vi "XW_Type_1b_correction.vi"(1 "variable n":bool, 2 "wire diameter (mu.m)":dbl, 3 "calib consts. t2":dbl[](array[numeric]), 4 "calib consts. t1":dbl[](array[numeric])) -> (0 "Corrected calib consts. t2":dbl[](array[numeric]))   [LabVIEW 2011]
panel:
  # "Type 1b: Correct calibration constants at t2 to conditions at t1"
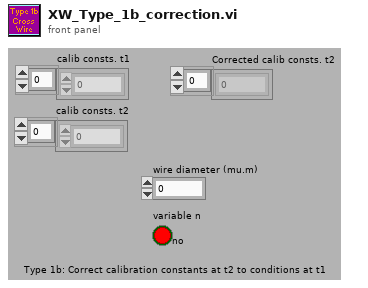
[diagram p1: front panel]
types:
  T1 = cluster{"calib consts. t1[0]":dbl, "calib consts. t1[1]":dbl, "calib consts. t1[2]":dbl, "calib consts. t1[3]":dbl, "calib consts. t1[4]":dbl, "calib consts. t1[5]":dbl, "calib consts. t1[6]":dbl, "calib consts. t1[7]":dbl, "calib consts. t1[8]":dbl, "calib consts. t1[9]":dbl, "calib consts. t1[10]":dbl, "calib consts. t1[11]":dbl, "calib consts. t1[12]":dbl, "calib consts. t1[13]":dbl, "calib consts. t1[14]":dbl, "calib consts. t1[15]":dbl, "calib consts. t1[16]":dbl, "calib consts. t1[17]":dbl}
  T2 = cluster{"calib consts. t2[0]":dbl, "calib consts. t2[1]":dbl, "calib consts. t2[2]":dbl, "calib consts. t2[3]":dbl, "calib consts. t2[4]":dbl, "calib consts. t2[5]":dbl, "calib consts. t2[6]":dbl, "calib consts. t2[7]":dbl, "calib consts. t2[8]":dbl, "calib consts. t2[9]":dbl, "calib consts. t2[10]":dbl, "calib consts. t2[11]":dbl, "calib consts. t2[12]":dbl, "calib consts. t2[13]":dbl, "calib consts. t2[14]":dbl, "calib consts. t2[15]":dbl, "calib consts. t2[16]":dbl, "calib consts. t2[17]":dbl}
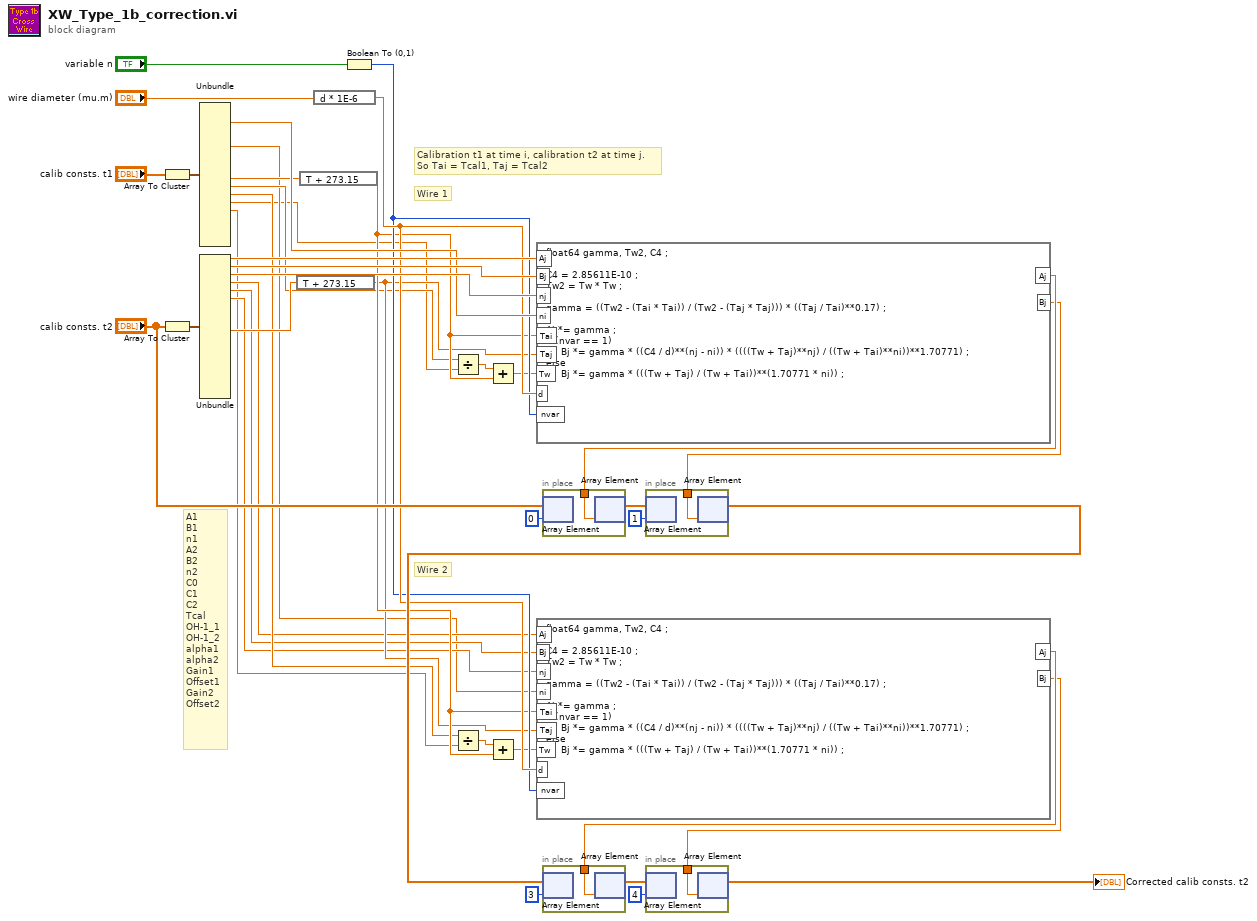
[diagram p0: block diagram]
diagram:
  # "Wire 2"
  # "Wire 1"
  # "A1\nB1\nn1\nA2\nB2\nn2\nC0\nC1\nC2\nTcal\nOH-1_1\nOH-1_2\nalpha1\nalpha2\nGain1\nOffset1\nGain2\nOffset2"
  # "Calibration t1 at time i, calibration t2 at time j.\nSo Tai = Tcal1, Taj = Tcal2"
  n1 = Array To Cluster(array="calib consts. t1") -> (cluster=w35:T1)
  n2 = Array To Cluster(array="calib consts. t2") -> (cluster=w40:T2)
  n3 = Unbundle(w35) -> ("calib consts. t1[2]"=w33:dbl, "calib consts. t1[5]"=w17:dbl, "calib consts. t1[9]"=w28:dbl, "calib consts. t1[10]"=w22:dbl, "calib consts. t1[11]"=w21:dbl, "calib consts. t1[12]"=w2:dbl, "calib consts. t1[13]"=w1:dbl)  [unwired: 11 out]
  n4 = Unbundle(w40) -> ("calib consts. t2[0]"=w39:dbl, "calib consts. t2[1]"=w38:dbl, "calib consts. t2[2]"=w37:dbl, "calib consts. t2[3]"=w20:dbl, "calib consts. t2[4]"=w19:dbl, "calib consts. t2[5]"=w18:dbl, "calib consts. t2[9]"=w27:dbl)  [unwired: 11 out]
  n5 = expression code="T + 273.15"(w27) -> (w23:dbl)
  n6 = expression code="T + 273.15"(w28) -> (w24:dbl)
  n7 = expression code="d * 1E-6"("wire diameter (mu.m)") -> (w26:dbl)
  n8 = Boolean To (0,1)(Boolean="variable n") -> (0, 1=w25:i16)
  n9 = Divide(x=w22, y=w2) -> (x/y=w16:dbl)
  n10 = Divide(x=w21, y=w1) -> (x/y=w9:dbl)
  n11 = Add(x=w16, y=w24) -> (x+y=w15:dbl)
  n12 = Add(x=w9, y=w24) -> (x+y=w8:dbl)
  n13 = formula code="float64 gamma, Tw2, C4 ;\n\nC4 = 2.85611E-10 ;\nTw2 = Tw * Tw ;\n\ngamma = ((Tw2 - (Tai * Tai)) / (Tw2 - (Taj * Taj))) * ((Taj / Tai)**0.17) ;\n\nAj *= gamma ;\nif (nvar == 1)\n     Bj *= gamma * ((C4 / d)**(nj - ni)) * ((((Tw + Taj)**nj) / ((Tw + Tai)**ni))**1.70771) ;\nelse\n     Bj *= gamma * (((Tw + Taj) / (Tw + Tai))**(1.70771 * ni)) ;"("Aj"=w39, "Bj"=w38, "nj"=w37, "Tai"=w24, "Taj"=w23, "Tw"=w15, "ni"=w33, "d"=w26, "nvar"=w25) -> ("Aj"=w13:dbl, "Bj"=w12:dbl)
  n14 = formula code="float64 gamma, Tw2, C4 ;\n\nC4 = 2.85611E-10 ;\nTw2 = Tw * Tw ;\n\ngamma = ((Tw2 - (Tai * Tai)) / (Tw2 - (Taj * Taj))) * ((Taj / Tai)**0.17) ;\n\nAj *= gamma ;\nif (nvar == 1)\n     Bj *= gamma * ((C4 / d)**(nj - ni)) * ((((Tw + Taj)**nj) / ((Tw + Tai)**ni))**1.70771) ;\nelse\n     Bj *= gamma * (((Tw + Taj) / (Tw + Tai))**(1.70771 * ni)) ;"("Aj"=w20, "Bj"=w19, "nj"=w18, "Tai"=w24, "Taj"=w23, "Tw"=w8, "ni"=w17, "d"=w26, "nvar"=w25) -> ("Aj"=w6:dbl, "Bj"=w5:dbl)
  n15 = in-place {
    in-place-border: w13 -> [w41]
    n16 = in-place-array #1("calib consts. t2", 0) -> ()  [unwired: 1 out]
    n17 = in-place-array #1(w41) -> (w10:dbl[])  [unwired: 1 out]
  }
  n18 = in-place {
    in-place-border: w12 -> [w42]
    n19 = in-place-array #2(w10, 1) -> ()  [unwired: 1 out]
    n20 = in-place-array #2(w42) -> (w30:dbl[])  [unwired: 1 out]
  }
  n21 = in-place {
    in-place-border: w6 -> [w43]
    n22 = in-place-array #3(w30, 3) -> ()  [unwired: 1 out]
    n23 = in-place-array #3(w43) -> (w3:dbl[])  [unwired: 1 out]
  }
  n24 = in-place {
    in-place-border: w5 -> [w44]
    n25 = in-place-array #4(w3, 4) -> ()  [unwired: 1 out]
    n26 = in-place-array #4(w44) -> (→"Corrected calib consts. t2":dbl[])  [unwired: 1 out]
  }
